vi "GetCustomProperties.vi"(11 "Properties":T2[](array[typedef])) -> (2 "Tdms Properties":T1[](array[typedef]))   [LabVIEW 2017, in "Tdms.lvlib"]
uses:
  <vilib>/addons/InsightCM/Utilities/Tdms/Tdms.lvlib
  <vilib>/addons/InsightCM/MessageBus/Base/controls/KeyValuePair.ctl
  <vilib>/addons/InsightCM/Utilities/Tdms/controls/Property.ctl
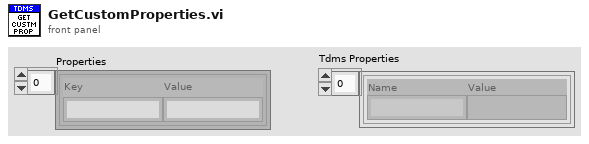
[diagram p1: front panel]
types:
  T1 = typedef "Tdms.lvlib/Property.ctl" = cluster{"Name":string, "Value":variant}
  T2 = typedef "KeyValuePair.ctl" = cluster{"Key":string, "Value":string}
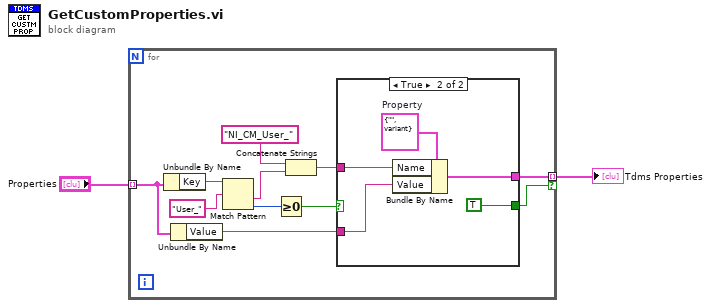
[diagram p0: block diagram]
diagram:
  n1 = for {
    tunnel: "Properties" -> [w9] mode=indexing
    tunnel: [w4] -> w1 mode=indexing if=w3
    n2 = Unbundle By Name(w9) -> ("Key"=w10:string)
    n3 = Unbundle By Name(w9) -> ("Value"=w8:string)
    n4 = Match Pattern(string=w10, regular expression="User_") -> (after substring=w6:string, offset past match=w13:i32)  [unwired: 1 in, 2 out]
    n5 = Greater Or Equal To 0?(x=w13) -> (x >= 0?=w11:bool)
    n6 = Concatenate Strings("NI_CM_User_" ("string"), w6) -> (w5:string)
    n7 = case shown="True" w11 {
      tunnel: w8 -> [_ w16]
      tunnel: w5 -> [_ w17]
      tunnel: [_ w15] -> w4
      tunnel: [_ TRUE] -> w3
      frame False {
      }
      frame True {
        w18 = T1 {"Name"="", "Value"=variant}  # Property
        n8 = Bundle By Name(cluster=w18, "Name"=w17, "Value"=w16) -> (w15:T1)
      }
    }
  }
  "Tdms Properties" <- w1
